vi "ReceiveJson.vi"(8 "error in (no error)":errorcluster, 10 "timeout [ms]":i32=5000, 11 "Communicator in":refnum<class "Communicator.lvclass">) -> (0 "error out":errorcluster, 2 "Data":string, 3 "Communicator out":refnum<class "Communicator.lvclass">)   [LabVIEW 2023, in "Communicator.lvclass"]
uses:
  Communicator.lvclass
  Communicator.lvclass/Communicator.ctl
  <vilib>/MediaMongrels Ltd/WebSockets/WebSockets/WebSocket Client/WebSocket Client.lvclass
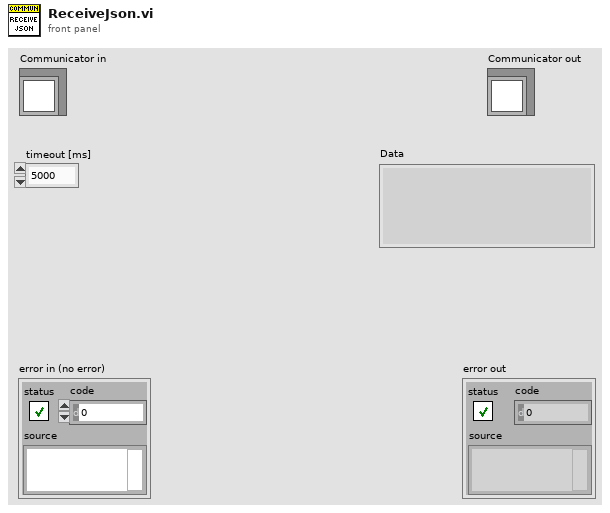
[diagram p1: front panel]
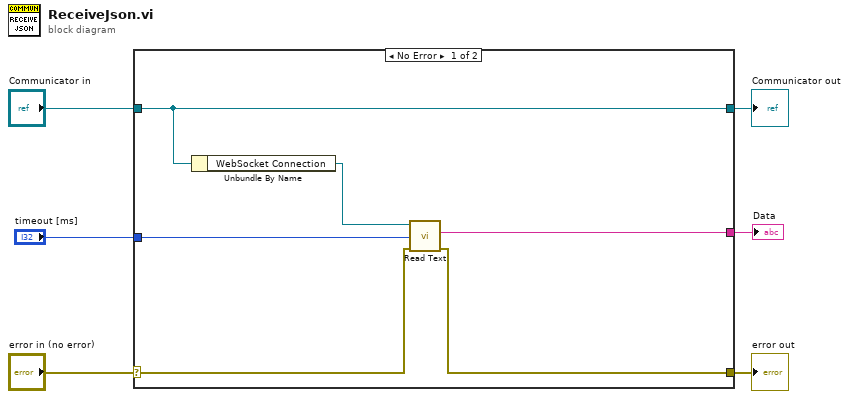
[diagram p0: block diagram]
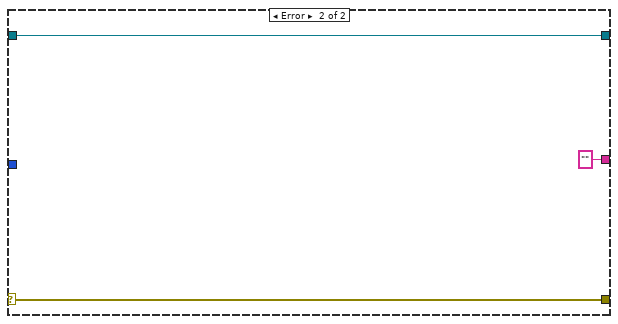
[diagram p2: hidden frame]
diagram:
  n1 = case shown="No Error" "error in (no error)" {
    selector: "error in (no error)" -> [w12 w15]
    tunnel: [w11 w15] -> w5
    tunnel: [w10 w14] -> w3
    tunnel: "Communicator in" -> [w10 w14]
    tunnel: "timeout [ms]" -> [w8 _]
    tunnel: [w7 "" ("Data")] -> w1
    frame No Error {
      n2 = Unbundle By Name(w10) -> ("WebSocket Connection"=w9:refnum<class "WebSocket Client.lvclass">)
      n3 = call-dynamic "Read Text.vi"("error in (no error)"=w12, "timeout ms (5000)"=w8, "WebSocket in"=w9) -> ("error out"=w11:errorcluster, "Data"=w7:string)  [unwired: 6 in, 1 out]
    }
    frame Error {
    }
  }
  "error out" <- w5
  "Communicator out" <- w3
  "Data" <- w1
